vi "Channel Selection.vi"(8 "error in (no error)":errorcluster, 10 "Number list":string, 11 "Red Pitaya Digitizer in":refnum<class "Red Pitaya Digitizer.lvclass">) -> (0 "error out":errorcluster, 1 "Boolean selection 2D":bool[][](array[boolean]), 2 "Selection":T1[](array[typedef]), 3 "Red Pitaya Digitizer out":refnum<class "Red Pitaya Digitizer.lvclass">, 4 "Boolean selection 1D":bool[](array[boolean]))   [LabVIEW 2024, in "Red Pitaya Digitizer.lvclass"]
uses:
  Red Pitaya Digitizer.lvclass
  Controls/Record Channels.ctl
  Red Pitaya Digitizer.lvclass/Red Pitaya Digitizer.ctl
  Read RP Instrument.vi
  RP Core/RP Instrument/RP Instrument.lvclass
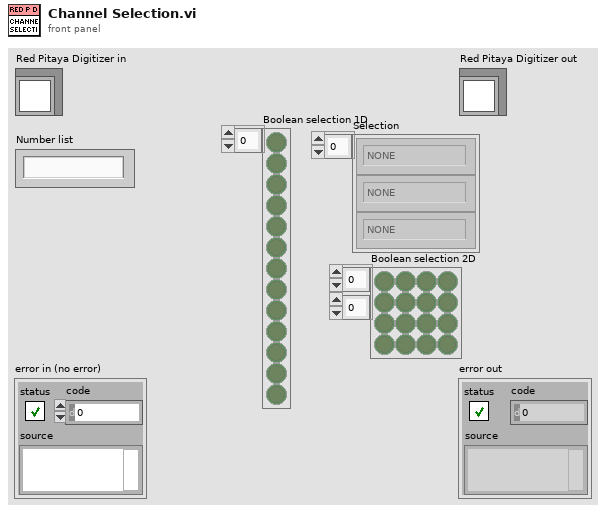
[diagram p1: front panel]
types:
  T1 = typedef "Record Channels.ctl" = enum16{"NONE", "FIRST", "SECOND", "BOTH"}
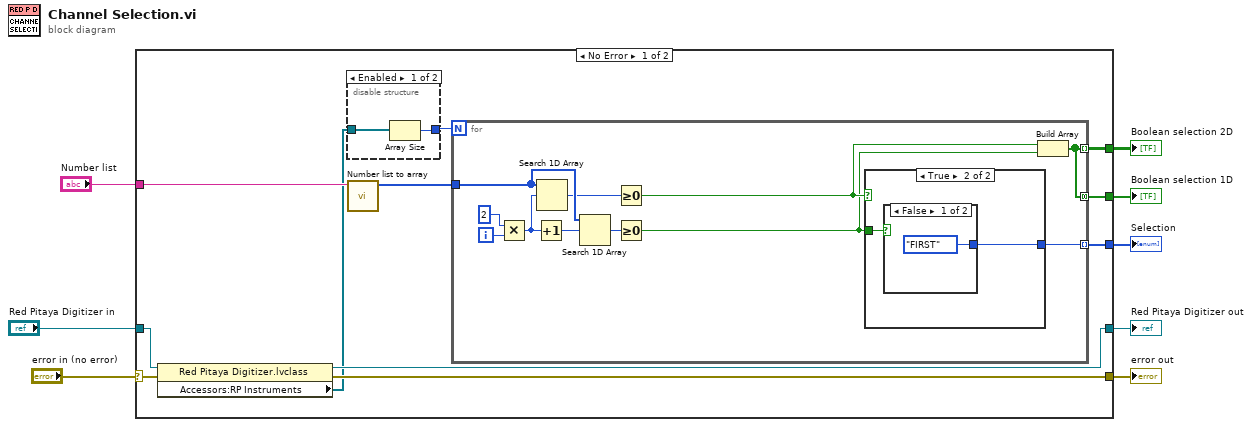
[diagram p0: block diagram]
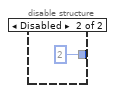
[diagram p2: hidden frame]
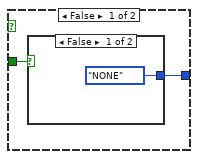
[diagram p3: hidden frame]
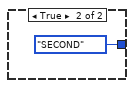
[diagram p4: hidden frame]
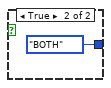
[diagram p5: hidden frame]
diagram:
  n1 = case shown="No Error" "error in (no error)" {
    selector: "error in (no error)" -> [w19 w43]
    tunnel: [w12 w43] -> w7
    tunnel: [w14 w42] -> w5
    tunnel: "Red Pitaya Digitizer in" -> [w13 w42]
    tunnel: "Number list" -> [w16 _]
    tunnel: [w15 _] -> w3
    tunnel: [w11 _] -> w2
    tunnel: [w10 _] -> w1
    frame No Error {
      n2 = property class="Red Pitaya Digitizer.lvclass"(reference=w13, error in=w19) -> (reference out=w14:refnum<class "Red Pitaya Digitizer.lvclass">, error out=w12:errorcluster, "Accessors:RP Instruments"=w9:refnum<class "RP Instrument.lvclass">[])
      n3 = disable-structure shown="Enabled" {
        disable-tunnel: [w21 2] -> w17
        disable-tunnel: w9 -> [w20 _]
        frame Enabled {
          n4 = Array Size(array=w20) -> (size(s)=w21:i32)
        }
        frame Disabled {
        }
      }
      n5 = call "Number list to array.vi"("Number list"=w16) -> ("Number list array"=w18:i32[])  [unwired: 8 in, 2 out]
      n6 = for {
        N: w17 -> [_]
        tunnel: w18 -> [w31]
        tunnel: [w28] -> w15 mode=indexing
        tunnel: [w23] -> w11 mode=indexing
        tunnel: [w23] -> w10 mode=concatenating
        i -> [w33]
        n7 = Multiply(x=2, y=w33) -> (x*y=w27:i32)
        n8 = Increment(x=w27) -> (x+1=w26:i32)
        n9 = Search 1D Array(1D array=w31, element=w27) -> (index of element=w30:i32)  [unwired: 1 in]
        n10 = Search 1D Array(1D array=w31, element=w26) -> (index of element=w29:i32)  [unwired: 1 in]
        n11 = Greater Or Equal To 0?(x=w30) -> (x >= 0?=w25:bool)
        n12 = Greater Or Equal To 0?(x=w29) -> (x >= 0?=w24:bool)
        n13 = case shown="True" w25 {
          tunnel: w24 -> [w35 w39]
          tunnel: [w34 w38] -> w28
          frame False {
            n14 = case shown="False" w35 {
              tunnel: [Record_Channels."NONE" Record_Channels."SECOND"] -> w34
              frame False {
              }
              frame True {
              }
            }
          }
          frame True {
            n15 = case shown="False" w39 {
              tunnel: [Record_Channels."FIRST" Record_Channels."BOTH"] -> w38
              frame False {
              }
              frame True {
              }
            }
          }
        }
        n16 = Build Array(w25, w24) -> (w23:bool[])
      }
    }
    frame Error {
    }
  }
  "error out" <- w7
  "Red Pitaya Digitizer out" <- w5
  "Selection" <- w3
  "Boolean selection 2D" <- w2
  "Boolean selection 1D" <- w1
